vi "Extract Newest Data.vi"(8 "Error":errorcluster, 9 "Name":refnum<class "_Pointer.lvclass">, 10 "Index":i32=-1, 11 "WavBuf":refnum<class "WavBuf.lvclass">) -> (0 "Error Out":errorcluster, 2 "Newest Data Out":T1, 3 "WavBuf Out":refnum<class "WavBuf.lvclass">)   [LabVIEW 2020, in "WavBuf.lvclass"]
uses:
  WavBuf.lvclass
  Universal Controls/Waveform_Data.ctl
  Pointer/_Pointer.lvclass
  WavBuf.lvclass/WavBuf.ctl
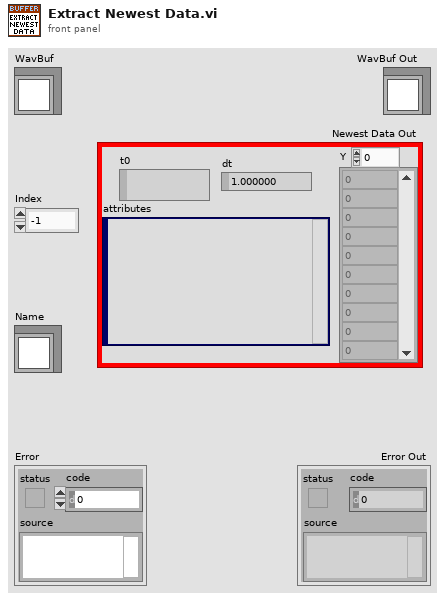
[diagram p1: front panel]
types:
  T1 = typedef "Waveform_Data.ctl" = waveform(dbl)
  T2 = typedef "Ref_DVR_Buffer.ctl" = refnum<data-value>
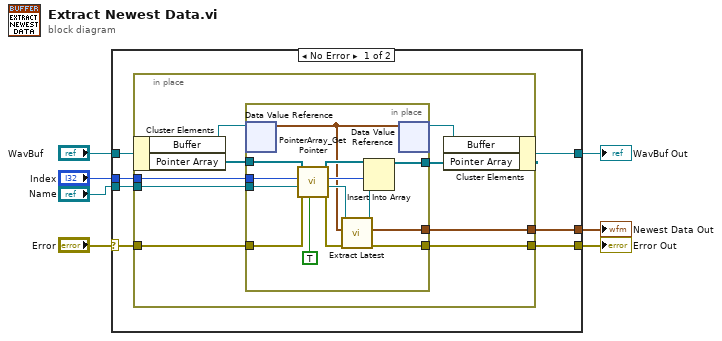
[diagram p0: block diagram]
diagram:
  n1 = case shown="No Error" "Error" {
    selector: "Error" -> [w12 w39]
    tunnel: [w11 w39] -> w6
    tunnel: [w13 w38] -> w4
    tunnel: "WavBuf" -> [w14 w38]
    tunnel: [w10 _] -> w3
    tunnel: "Name" -> [w9 _]
    tunnel: "Index" -> [w8 _]
    frame No Error {
      n2 = in-place {
        in-place-border: w12 -> [w23]
        in-place-border: [w18] -> w11
        in-place-border: [w17] -> w10
        in-place-border: w9 -> [w20]
        in-place-border: w8 -> [w19]
        n3 = in-place-cluster #1(w14) -> ("Buffer"=w16:T2, "Pointer Array"=w22:refnum<class "_Pointer.lvclass">[])
        n4 = in-place {
          in-place-border: w23 -> [w37]
          in-place-border: w22 -> [w35]
          in-place-border: [w33] -> w21
          in-place-border: w20 -> [w32]
          in-place-border: w19 -> [w31]
          in-place-border: [w28] -> w18
          in-place-border: [w25] -> w17
          n5 = in-place-dvr #2(w16) -> (w24:T1)  [unwired: 1 out]
          n6 = call "PointerArray_Get Pointer.vi"("Create If Not Found"=TRUE ("Create if not found"), "Error"=w37, "Pointer"=w32, "Index"=w31, "Pointer Array"=w35) -> ("Error Out"=w29:errorcluster, "Pointer Out"=w27:refnum<class "_Pointer.lvclass">, "Index Out"=w30:i32, "Pointer Array Out"=w36:refnum<class "_Pointer.lvclass">[])  [unwired: 2 in, 1 out]
          n7 = call-dynamic "Extract Latest.vi"("Error"=w29, "Raw Data Waveform"=w24, "((Pointer))"=w27) -> ("Error Out"=w28:errorcluster, "Waveform Out"=w25:T1, "((Pointer)) Out"=w26:refnum<class "_Pointer.lvclass">)  [unwired: 6 in]
          n8 = Insert Into Array(array=w36, index=w30, new element=w26) -> (w33:refnum<class "_Pointer.lvclass">[])
          n9 = in-place-dvr #2(w24) -> (w15:T2)  [unwired: 1 out]
        }
        n10 = in-place-cluster #1("Buffer"=w15, "Pointer Array"=w21) -> (w13:refnum<class "WavBuf.lvclass">)
      }
    }
    frame Error {
    }
  }
  "Error Out" <- w6
  "WavBuf Out" <- w4
  "Newest Data Out" <- w3
